vi "Header.CreateBroadcasts.vi"(8 "error in (no error)":errorcluster) -> (0 "error out":errorcluster, 3 "Broadcasts":T1)   [LabVIEW 2024, in "Header.lvclass"]
uses:
  Header.lvclass
  Broadcast Events--cluster.ctl
  Stopped.ctl
  Header.lvclass/Header.ctl
  JQMHCore/Module/RQMHModule.lvclass
  Menu Item Selected.ctl
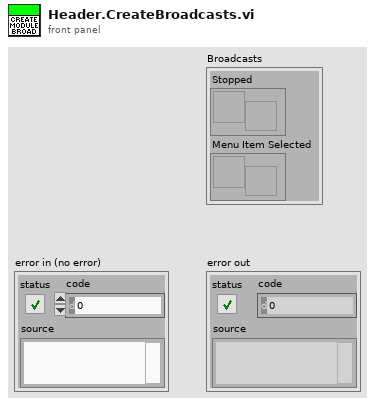
[diagram p1: front panel]
types:
  T1 = typedef "Header.lvclass/Broadcast Events--cluster.ctl" = cluster{"Stopped":refnum<user-event>, "Menu Item Selected":refnum<user-event>}
  T2 = typedef "Header.lvclass/Menu Item Selected.ctl" = cluster{"Module":refnum<class "RQMHModule.lvclass">, "Menu Item":string}
  T3 = typedef "Header.lvclass/Stopped.ctl" = bool
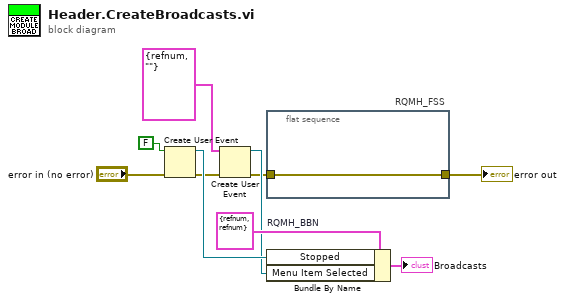
[diagram p0: block diagram]
diagram:
  n1 = Create User Event(user event datatype=T3 FALSE ("Stopped"), error in="error in (no error)") -> (user event=w9:refnum<user-event>, error out=w2:errorcluster)
  n2 = Create User Event(user event datatype=T2 {"Module"=refnum, "Menu Item"=""} ("Menu Item Selected"), error in=w2) -> (user event=w3:refnum<user-event>, error out=w1:errorcluster)
  n3 = flat-sequence "RQMH_FSS" {
    tunnel: w1 -> [w11]
    tunnel: [w11] -> w5
    frame #0 {
    }
  }
  n4 = Bundle By Name "RQMH_BBN"(cluster=T1 {"Stopped"=refnum, "Menu Item Selected"=refnum} ("Broadcasts"), "Stopped"=w9, "Menu Item Selected"=w3) -> (→"Broadcasts":T1)
  "error out" <- w5
